vi "LinearQuadraticRegulator_GetK_Single.vi"(9 "Row":i32, 11 "in LinearQuadraticRegulator":T1) -> (3 "K":dbl)   [LabVIEW 2019, in "Trajectory_Library.lvlib"]
doc: "Returns a single element of the controller matrix K.\n \nInput:\n - LinearQuadraticRegulator -- controller data cluster\n - row -- index into the row of K (0-n)\n\nOutputs:\n - K -- the controller single value K."
uses:
  Trajectory_Library.lvlib
  <vilib>/Analysis/Matrix/Datatypes/RealMatrix.ctl
  <vilib>/Analysis/Matrix/NI_Matrix.lvlib
  TypeDef/LINEAR_QUADRATIC_REGULATOR.ctl
panel:
  # "Ref State <States,1>"
  # "Comp and capped \noutput <Inputs,1>"
  # "Controller gain\n<Inputs,States>"
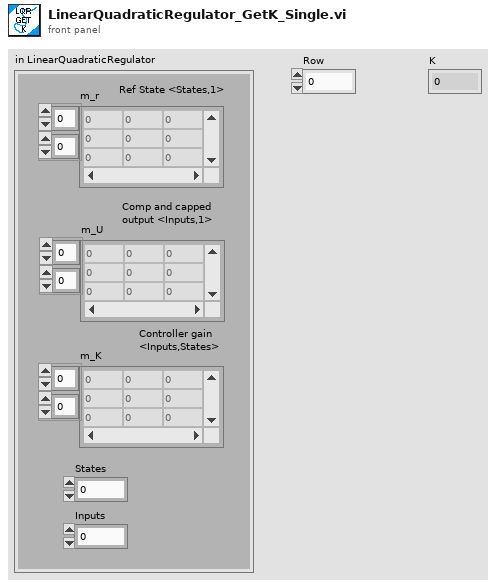
[diagram p1: front panel]
types:
  T1 = typedef "Trajectory_Library.lvlib/LINEAR_QUADRATIC_REGULATOR.ctl" = cluster{"m_r":T2, "m_U":T2, "m_K":T2, "States":i32, "Inputs":i32}
  T2 = typedef "NI_Matrix.lvlib/RealMatrix.ctl" = dbl[][]
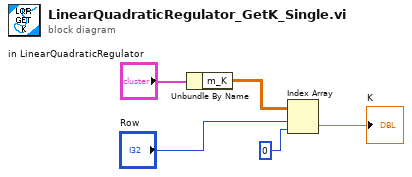
[diagram p0: block diagram]
diagram:
  n1 = Unbundle By Name("in LinearQuadraticRegulator") -> ("m_K"=w4:T2)
  n2 = Index Array(array=w4, index (row)="Row", index (col)=0) -> (element=→"K":dbl)
